vi "ResolveSymbolicPath.vi"(9 "Overwrite LabVIEW Folder(If empty use this version of LabVIEW)":path, 11 "path":path) -> (3 "File Path":path)   [LabVIEW 2020, in "DependencyChecker.lvlib"]
uses:
  DependencyChecker.lvlib
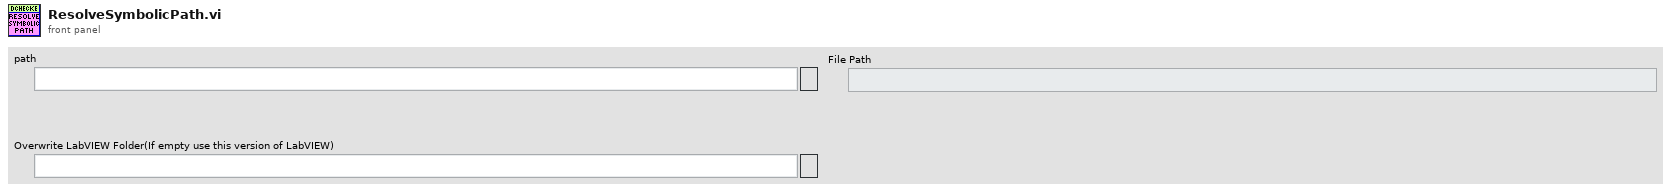
[diagram p1: front panel]
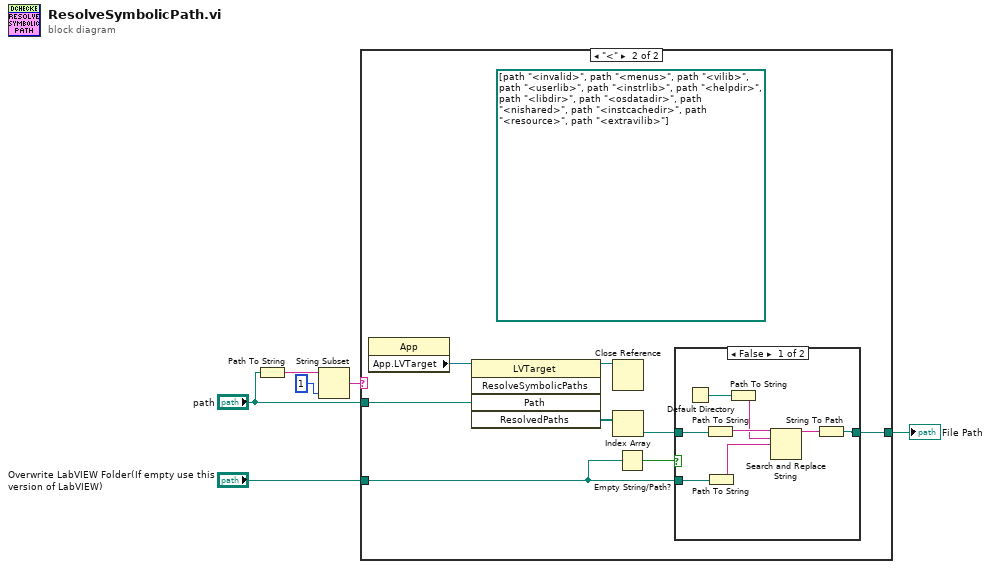
[diagram p0: block diagram]
diagram:
  n1 = Path To String(path="path") -> (string=w6:string)
  n2 = String Subset(string=w6, length (rest)=1 ("length (rest)")) -> (substring=w4:string)  [unwired: 1 in]
  n3 = case shown="\"<\"" w4 {
    tunnel: "path" -> [w7 w13]
    tunnel: [w7 w9] -> w2
    tunnel: "Overwrite LabVIEW Folder(If empty use this version of LabVIEW)" -> [_ w8]
    frame "False", Default {
    }
    frame "<" {
      (unwired) path[] [path "<invalid>", path "<menus>", path "<vilib>", path "<userlib>", path "<instrlib>", path "<helpdir>", path "<libdir>", path "<osdatadir>", path "<nishared>", path "<instcachedir>", path "<resource>", path "<extravilib>"]
      n4 = property class="App"() -> ("App.LVTarget"=w14:refnum<vi>)  [unwired: 2 in, 2 out]
      n5 = invoke class="LVTarget" method="ResolveSymbolicPaths"(reference=w14, "Path"=w13) -> (reference out=w15:refnum<vi>, "ResolvedPaths"=w12:path[])  [unwired: 3 in, 3 out]
      n6 = Close Reference(reference=w15) -> ()  [unwired: 1 in, 1 out]
      n7 = Index Array(array=w12) -> (element=w10:path)  [unwired: 1 in]
      n8 = Empty String/Path?(string/path=w8) -> (empty?=w11:bool)
      n9 = case shown="False" w11 {
        tunnel: w10 -> [w23 w24]
        tunnel: [w17 w24] -> w9
        tunnel: w8 -> [w20 _]
        frame False {
          n10 = Default Directory() -> (w16:path)
          n11 = Path To String(path=w23) -> (string=w22:string)
          n12 = Path To String(path=w20) -> (string=w19:string)
          n13 = Path To String(path=w16) -> (string=w21:string)
          n14 = Search and Replace String(input string=w22, search string=w21, replace string=w19) -> (result string=w18:string)  [unwired: 5 in, 3 out]
          n15 = String To Path(string=w18) -> (path=w17:path)
        }
        frame True {
        }
      }
    }
  }
  "File Path" <- w2
